vi "example.vi"() -> ()   [LabVIEW 2018]
uses:
  type.ctl
  MatFileLib.lvlib
panel:
  in  "FolderName":string
  out "Created":bool
  in  "file_name":string="name_file"
  out "error out":errorcluster
  in  "Contents":string[](array[string])=["arraynameA", "arraynameB", "arraynameC"]
  in  "Type":T1[](array[typedef])=[enum."Double64bit", enum."Double64bit_elem", enum."Int64bit"]
  in  "file path (use dialog)":path=path "E:/GruppoMisure/GiovanniDAvanzo/WorkSpace/ImekoTC10_2019/WorkspaceLabviewForPMU/MatFile"
  # "name file without .mat\nset content list and type of contents"
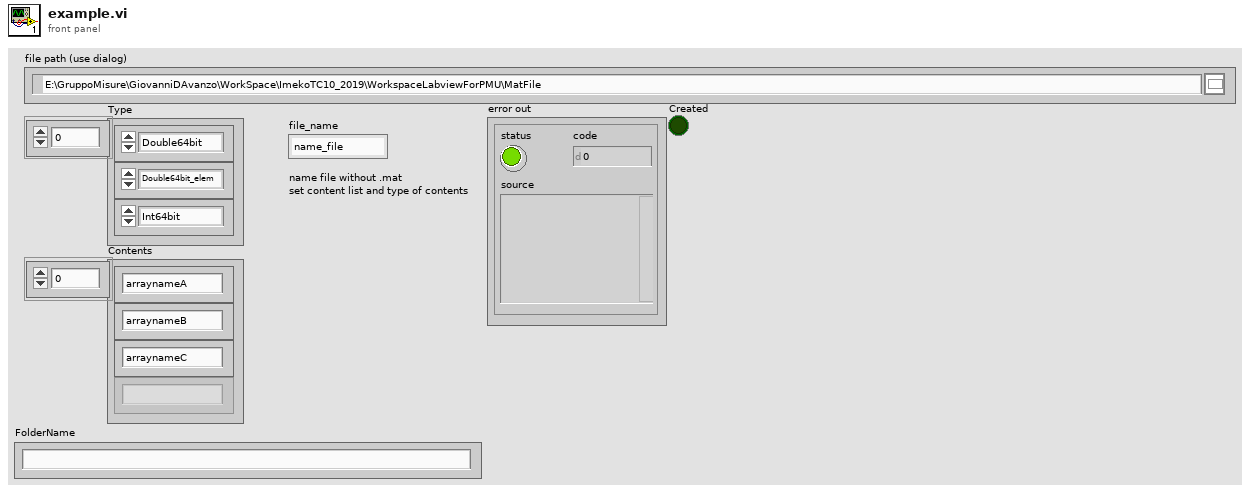
[diagram p1: front panel]
types:
  T1 = typedef "MatFileLib.lvlib/type.ctl" = enum16{"Int8bit_elem", "Int8bit", "Int64bit_elem", "Int64bit", "Int16bit_elem", "Double64bit_elem", "Int16bit", "Double64bit"}
  T2 = enum16{"open", "replace", "create", "open or create", "replace or create", "replace or create with confirmation"}
  T3 = typedef "MatFileLib.lvlib/matFile_info.ctl" = cluster{"file path (use dialog)":path, "refnum file":refnum<file>, "intermediate array":cluster{"intermediate":refnum<file>, "array name dim":i32, "row":i32, "col":i32, "Content":string, "Enum":T1}[]}
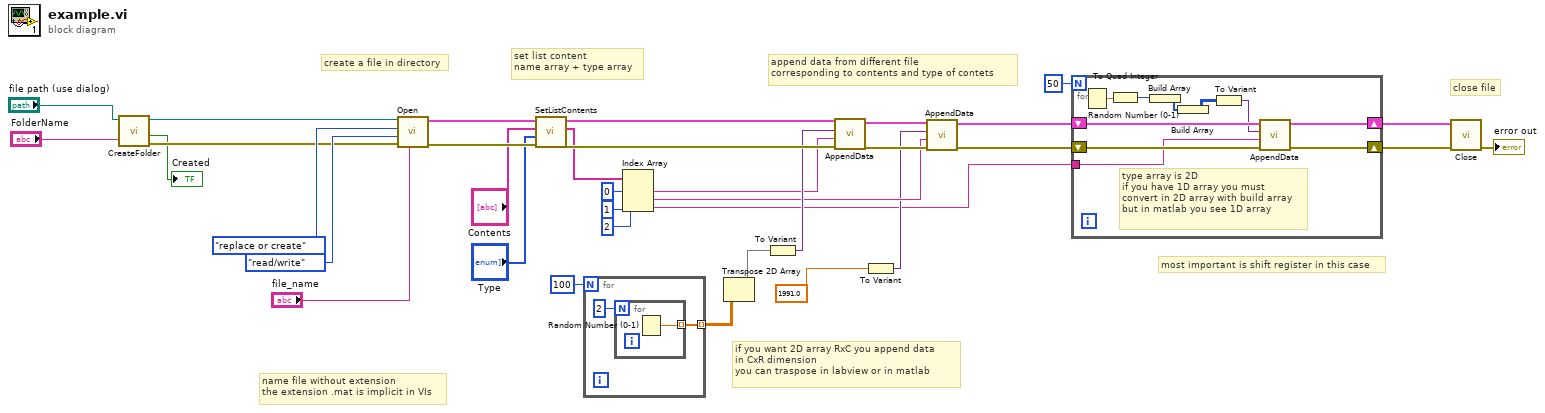
[diagram p0: block diagram]
diagram:
  # "if you want 2D array RxC you append data \nin CxR dimension\nyou can traspose in labview or in matlab"
  # "most important is shift register in this case"
  # "close file"
  # "append data from different file\ncorresponding to contents and type of contets"
  # "set list content\nname array + type array"
  # "create a file in directory"
  # "name file without extension\nthe extension .mat is implicit in VIs"
  n1 = call "CreateFolder.vi"("FolderName"="FolderName", "main path"="file path (use dialog)") -> ("error out"=w4:errorcluster, "Created"=→"Created":bool, "path out"=w3:path)  [unwired: 7 in]
  n2 = call "Open.vi"("file_name"="file_name", "error in"=w4, "access (0:read/write)"=enum16{"read/write", "read-only", "write-only"}."read/write", "operation (0:open)"=T2."replace or create", "file path (use dialog)"=w3) -> ("error out"=w31:errorcluster, "matFile_info"=w32:T3)  [unwired: 4 in]
  n3 = call "SetListContents.vi"("error in"=w31, "Type"="Type", "Contents"="Contents", "matFile_info IN"=w32) -> ("error out"=w27:errorcluster, "Contents"=w24:string[], "matFile_info OUT"=w28:T3)  [unwired: 5 in]
  n4 = for {
    N: 100 -> [_]
    tunnel: [w36] -> w17 mode=indexing
    n5 = for {
      N: 2 -> [_]
      tunnel: [w38] -> w36 mode=indexing
      n6 = Random Number (0-1)() -> (number: 0 to 1=w38:dbl)
    }
  }
  n7 = Index Array(array=w24, index #1=0 ("index"), index #2=1 ("index"), index #3=2 ("index")) -> (element #1=w22:string, element #2=w18:string, element #3=w13:string)
  n8 = Transpose 2D Array(2D array=w17) -> (transposed array=w6:dbl[][])
  n9 = To Variant(anything=w6) -> (Variant=w25:variant)
  n10 = call "AppendData.vi"("error in"=w27, "Content"=w22, "Variant"=w25, "matFile_info IN"=w28) -> ("error out"=w20:errorcluster, "matFile_info OUT"=w21:T3)  [unwired: 6 in]
  n11 = To Variant(anything=1991.0) -> (Variant=w16:variant)
  n12 = call "AppendData.vi"("error in"=w20, "Content"=w18, "Variant"=w16, "matFile_info IN"=w21) -> ("error out"=w15:errorcluster, "matFile_info OUT"=w9:T3)  [unwired: 6 in]
  n13 = for {
    N: 50 -> [_]
    tunnel: w13 -> [w47]
    shift-right: [w46] -> w12
    shift-left: w15 -> [w48]
    shift-right: [w45] -> w11
    shift-left: w9 -> [w44]
    # "type array is 2D \nif you have 1D array you must \nconvert in 2D array with build array\nbut in matlab you see 1D array"
    n14 = Random Number (0-1)() -> (number: 0 to 1=w43:dbl)
    n15 = To Quad Integer(1:w43) -> (0:w42:i64)
    n16 = Build Array(w42) -> (w40:i64[])
    n17 = Build Array(w40) -> (w39:i64[][])
    n18 = To Variant(anything=w39) -> (Variant=w41:variant)
    n19 = call "AppendData.vi"("error in"=w48, "Content"=w47, "Variant"=w41, "matFile_info IN"=w44) -> ("error out"=w46:errorcluster, "matFile_info OUT"=w45:T3)  [unwired: 6 in]
  }
  n20 = call "Close.vi"("error in"=w12, "matFile_info IN"=w11) -> ("error out"=→"error out":errorcluster)  [unwired: 8 in, 1 out]
